vi "APX TMP control.vi"() -> ()   [LabVIEW 2015]
uses:
  <vilib>/Instr/_visa.llb/VISA Configure Serial Port (Instr).vi
  <userlib>/caLab/Private/Get_PV-1D.vi
  <userlib>/caLab/Private/Put_DBL-1D_PV-1D.vi
panel:
  out "Status":bool
  in  "stop":bool
  in  "APX:BPTurebo_ENB":bool
  in  "APX:GASTurbo_ENB":bool
  in  "APX:HPCTurbo_ENB":bool
  in  "APX:PREPTurbo_ENB":bool
  in  "APX:HEMTurbo_ENB":bool
  in  "APX:L2Turbo_ENB":bool
  in  "APX:AP2Turbo_ENB":bool
  in  "APX:AP1Turbo_ENB":bool
  out "APX:BPTurboS":dbl
  out "APX:BPTrubo_STOP":bool
  out "APX:BPTurbo_START":bool
  out "APX:BPTurboPort":refnum<visa-resource-name>="COM4"
  out "APX:BPTurboF":dbl caption="F_20/Hz"
  out "APX:BPTurboP":dbl caption="P_20/W"
  out "APX:BPTurboS:STR":string
  out "APX:GASTurboS":dbl
  out "APX:GASTurbo_STOP":bool
  out "APX:GASTurbo_START":bool
  out "APX:GASTurboPort":refnum<visa-resource-name>="COM4"
  out "APX:GASTurboF":dbl caption="F_20/Hz"
  out "APX:GASTurboP":dbl caption="P_20/W"
  out "APX:GASTurboS:STR":string
  out "APX:HPCTurboS":dbl
  out "APX:HPCTrubo_STOP":bool
  out "APX:HPCTurbo_START":bool
  out "APX:HPCTurboPort":refnum<visa-resource-name>="COM4"
  out "APX:HPCTurboF":dbl caption="F_20/Hz"
  out "APX:HPCTurboP":dbl caption="P_20/W"
  out "APX:HPCTurboS:STR":string
  out "APX:PREPTurboS":dbl
  out "APX:PREPTrubo_STOP":bool
  out "APX:PREPTurbo_START":bool
  out "APX:PREPTurboPort":refnum<visa-resource-name>="COM4"
  out "APX:PREPTurboF":dbl caption="F_20/Hz"
  out "APX:PREPTurboP":dbl caption="P_20/W"
  out "APX:PREPTurboS:STR":string
  out "APX:HEMTurboS":dbl
  out "APX:HEMTrubo_STOP":bool
  out "APX:HEMTurbo_START":bool
  out "APX:HEMTurboPort":refnum<visa-resource-name>="COM4"
  out "APX:HEMTurboF":dbl caption="F_20/Hz"
  out "APX:HEMTurboP":dbl caption="P_20/W"
  out "APX:HEMTurboS:STR":string
  out "APX:L2TurboS":dbl
  out "APX:L2Trubo_STOP":bool
  out "APX:L2Turbo_START":bool
  out "APX:L2TuroboPort":refnum<visa-resource-name>="COM4"
  out "APX:L2TurboF":dbl caption="F_20/Hz"
  out "APX:L2TurboP":dbl caption="P_20/W"
  out "APX:L2STurboS:STR":string
  out "APX:AP2TurboS":dbl
  out "APX:AP2Trubo_STOP":bool
  out "APX:AP2Turbo_START":bool
  out "APX:AP2TruboPort":refnum<visa-resource-name>="COM4"
  out "APX:AP2TurboF":dbl caption="F_20/Hz"
  out "APX:AP2TurboP":dbl caption="P_20/W"
  out "APX:AP2TurboS:STR":string
  out "APX:AP1STurboS":dbl
  out "APX:AP1Trubo_STOP":bool
  out "APX:APITurbo_START":bool
  out "APX:AP1TurboPort":refnum<visa-resource-name>="COM4"
  out "APX:AP1TurboF":dbl caption="F_20/Hz"
  out "APX:AP1TurboP":dbl caption="P_20/W"
  out "APX:AP1TurboS:STR":string
  # "APX Turbo"
  # "COM6"
  # "COM4"
  # "COM5"
  # "COM25"
  # "COM26"
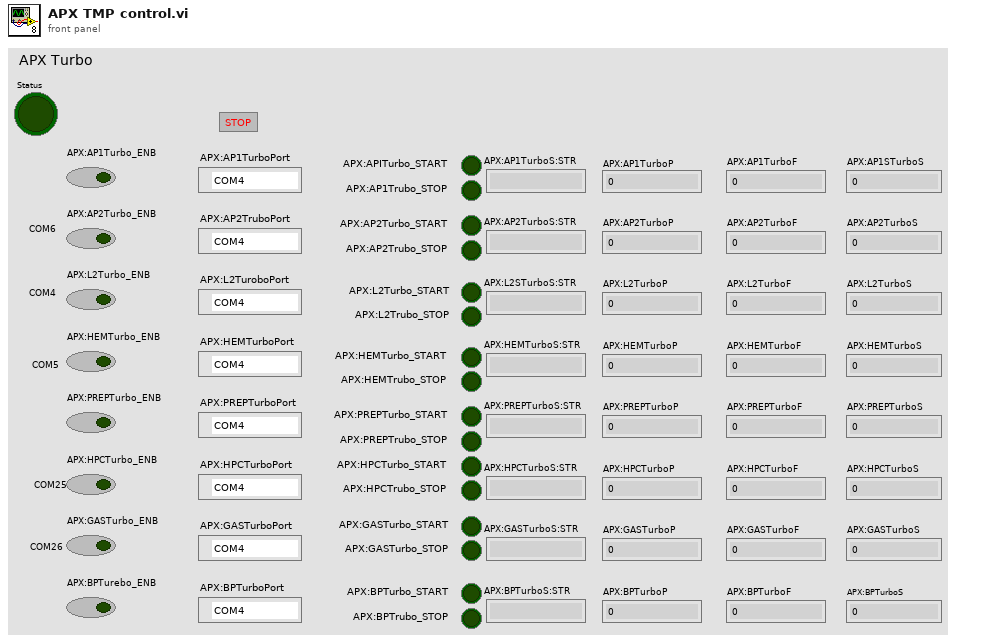
[diagram p1: front panel]
types:
  T1 = enum16{"START", "STOP", "REMOTE/SERIAL", "REMOTE", "SERIAL", "START/STOP", "PUMP STATUS", "Driving Frequency", "PUMP POWER", "PRESSURE"}
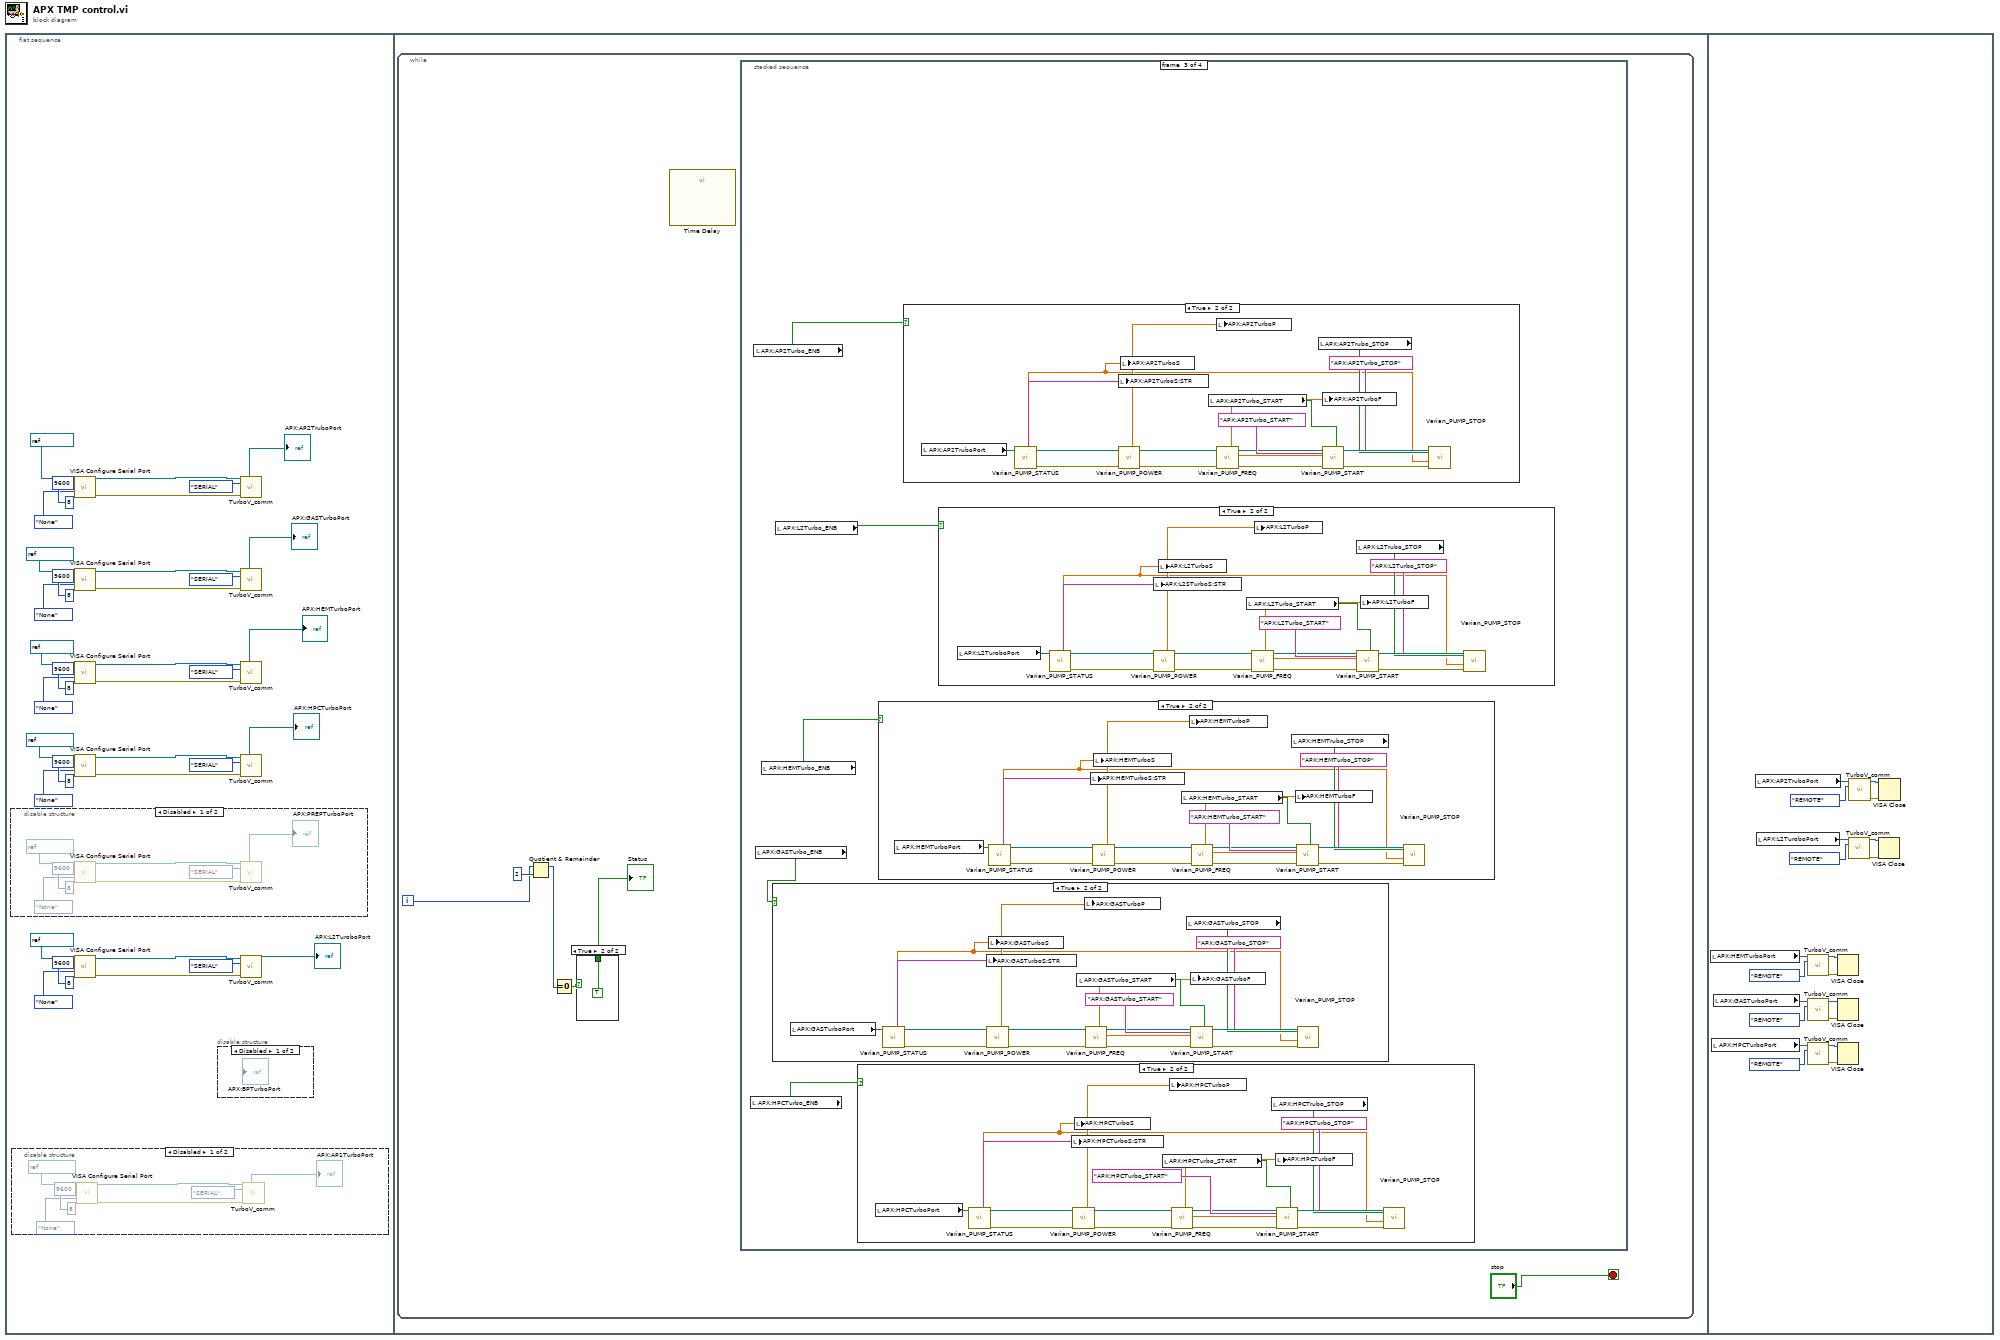
[diagram p0: block diagram]
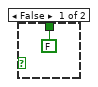
[diagram p5: hidden frame]
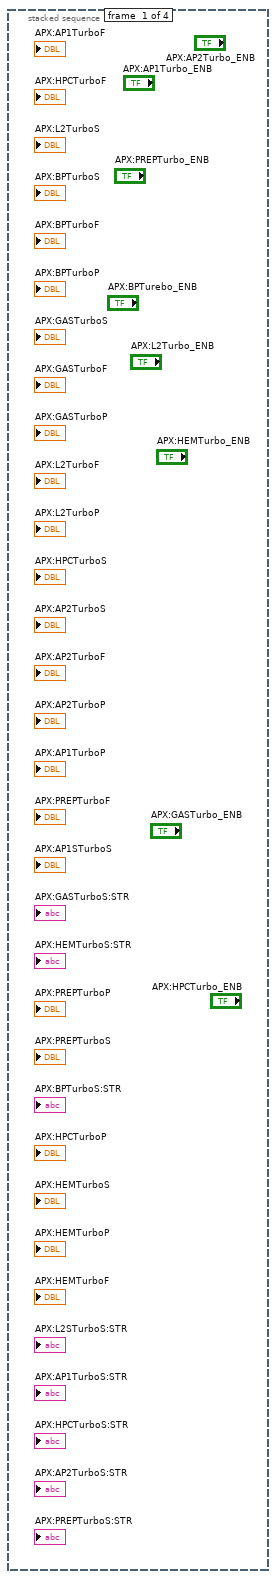
[diagram p6: hidden frame]
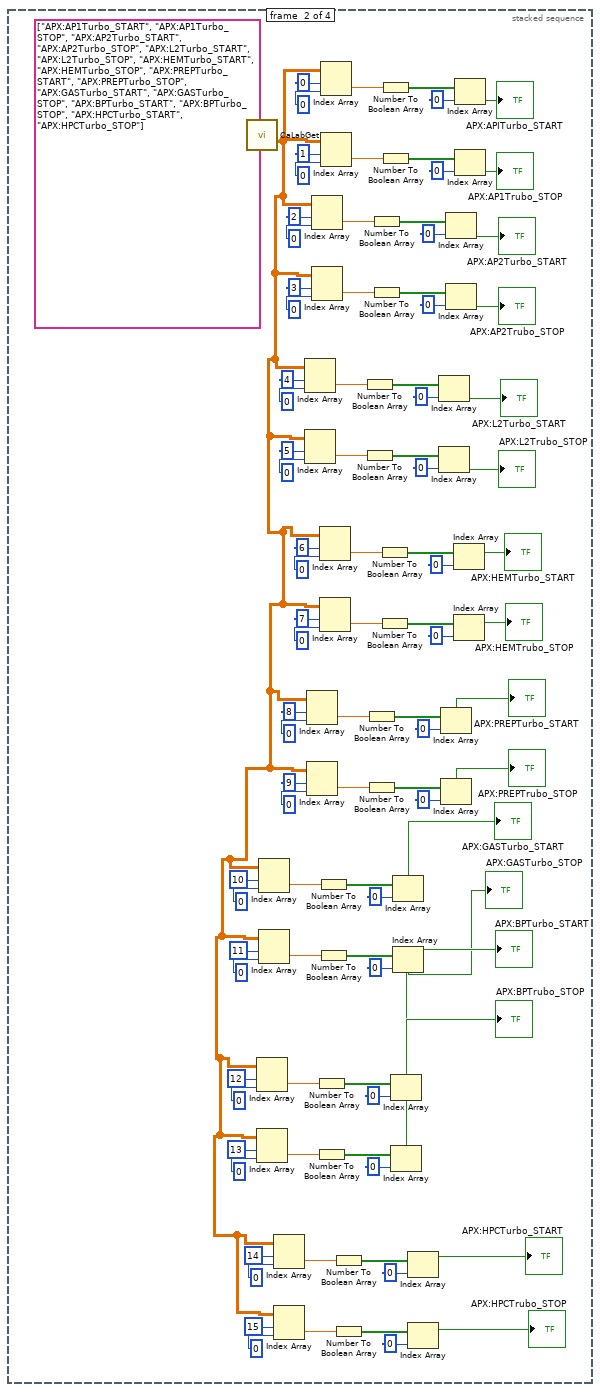
[diagram p7: hidden frame]
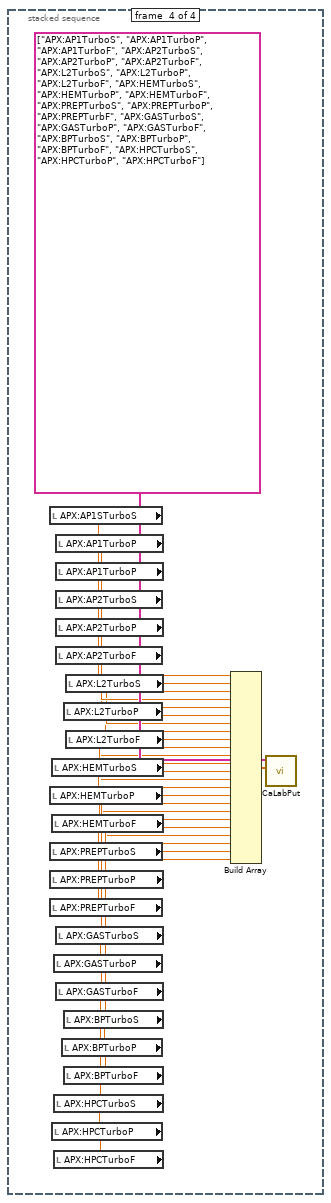
[diagram p13: hidden frame]
diagram:
  n1 = flat-sequence {
    frame #0 {
      n2 = disable-structure shown="Disabled" {
        frame Disabled {
          n3 = call-poly "VISA Configure Serial Port"("VISA resource name"=refnum<visa-resource-name> "COM26", "baud rate (9600)"=u32 9600, "data bits (8)"=u16 8, "parity (0:none)"=enum16{"None", "Odd", "Even", "Mark", "Space"}."None") -> ("VISA resource name out"=w53:refnum<visa-resource-name>, "error out"=w52:errorcluster)  [unwired: 10 in]
          n4 = call "TurboV_comm.vi"("VISA resource name"=w53, "Command"=T1."SERIAL", "error in (no error)"=w52) -> ("VISA resource name out"=→"APX:PREPTurboPort":refnum<visa-resource-name>)  [unwired: 10 in, 2 out]
        }
        frame Enabled {
        }
      }
      n5 = disable-structure shown="Disabled" {
        frame Disabled {
          n6 = call-poly "VISA Configure Serial Port"("VISA resource name"=refnum<visa-resource-name> "COM26", "baud rate (9600)"=u32 9600, "data bits (8)"=u16 8, "parity (0:none)"=enum16{"None", "Odd", "Even", "Mark", "Space"}."None") -> ("VISA resource name out"=w44:refnum<visa-resource-name>, "error out"=w43:errorcluster)  [unwired: 10 in]
          n7 = call "TurboV_comm.vi"("VISA resource name"=w44, "Command"=T1."SERIAL", "error in (no error)"=w43) -> ("VISA resource name out"=→"APX:AP1TurboPort":refnum<visa-resource-name>)  [unwired: 10 in, 2 out]
        }
        frame Enabled {
        }
      }
      n8 = call-poly "VISA Configure Serial Port"("VISA resource name"=refnum<visa-resource-name> "COM6", "baud rate (9600)"=u32 9600, "data bits (8)"=u16 8, "parity (0:none)"=enum16{"None", "Odd", "Even", "Mark", "Space"}."None") -> ("VISA resource name out"=w9:refnum<visa-resource-name>, "error out"=w8:errorcluster)  [unwired: 10 in]
      n9 = call-poly "VISA Configure Serial Port"("VISA resource name"=refnum<visa-resource-name> "COM26", "baud rate (9600)"=u32 9600, "data bits (8)"=u16 8, "parity (0:none)"=enum16{"None", "Odd", "Even", "Mark", "Space"}."None") -> ("VISA resource name out"=w16:refnum<visa-resource-name>, "error out"=w15:errorcluster)  [unwired: 10 in]
      n10 = call-poly "VISA Configure Serial Port"("VISA resource name"=refnum<visa-resource-name> "COM5", "baud rate (9600)"=u32 9600, "data bits (8)"=u16 8, "parity (0:none)"=enum16{"None", "Odd", "Even", "Mark", "Space"}."None") -> ("VISA resource name out"=w23:refnum<visa-resource-name>, "error out"=w22:errorcluster)  [unwired: 10 in]
      n11 = call-poly "VISA Configure Serial Port"("VISA resource name"=refnum<visa-resource-name> "COM25", "baud rate (9600)"=u32 9600, "data bits (8)"=u16 8, "parity (0:none)"=enum16{"None", "Odd", "Even", "Mark", "Space"}."None") -> ("VISA resource name out"=w30:refnum<visa-resource-name>, "error out"=w29:errorcluster)  [unwired: 10 in]
      n12 = call-poly "VISA Configure Serial Port"("VISA resource name"=refnum<visa-resource-name> "COM4", "baud rate (9600)"=u32 9600, "data bits (8)"=u16 8, "parity (0:none)"=enum16{"None", "Odd", "Even", "Mark", "Space"}."None") -> ("VISA resource name out"=w37:refnum<visa-resource-name>, "error out"=w36:errorcluster)  [unwired: 10 in]
      n13 = disable-structure shown="Disabled" {
        frame Disabled {
        }
        frame Enabled {
        }
      }
      n14 = call "TurboV_comm.vi"("VISA resource name"=w9, "Command"=T1."SERIAL", "error in (no error)"=w8) -> ("VISA resource name out"=→"APX:AP2TruboPort":refnum<visa-resource-name>)  [unwired: 10 in, 2 out]
      n15 = call "TurboV_comm.vi"("VISA resource name"=w16, "Command"=T1."SERIAL", "error in (no error)"=w15) -> ("VISA resource name out"=→"APX:GASTurboPort":refnum<visa-resource-name>)  [unwired: 10 in, 2 out]
      n16 = call "TurboV_comm.vi"("VISA resource name"=w23, "Command"=T1."SERIAL", "error in (no error)"=w22) -> ("VISA resource name out"=→"APX:HEMTurboPort":refnum<visa-resource-name>)  [unwired: 10 in, 2 out]
      n17 = call "TurboV_comm.vi"("VISA resource name"=w30, "Command"=T1."SERIAL", "error in (no error)"=w29) -> ("VISA resource name out"=→"APX:HPCTurboPort":refnum<visa-resource-name>)  [unwired: 10 in, 2 out]
      n18 = call "TurboV_comm.vi"("VISA resource name"=w37, "Command"=T1."SERIAL", "error in (no error)"=w36) -> ("VISA resource name out"=→"APX:L2TuroboPort":refnum<visa-resource-name>)  [unwired: 10 in, 2 out]
    }
    frame #1 {
      n19 = while {
        i -> [w58]
        stop <- "stop" stop-if-true
        n20 = Quotient & Remainder(x=w58, y=2) -> (x-y*floor(x/y)=w60:i32)  [unwired: 1 out]
        n21 = Equal To 0?(x=w60) -> (x = 0?=w61:bool)
        n22 = case shown="True" w61 {
          tunnel: [FALSE ("Status") TRUE ("Status")] -> w57
          frame False {
          }
          frame True {
          }
        }
        "Status" <- w57
        n23 = call "Time Delay"() -> ()  [unwired: 11 in, 1 out]
        n24 = stacked-sequence {
          frame #0 {
          }
          frame #1 {
            n25 = call-poly "CaLabGet.vi"("PV Names"=string[] ["APX:AP1Turbo_START", "APX:AP1Turbo_STOP", "APX:AP2Turbo_START", "APX:AP2Turbo_STOP", "APX:L2Turbo_START", "APX:L2Turbo_STOP", "APX:HEMTurbo_START", "APX:HEMTurbo_STOP", "APX:PREPTurbo_START", "APX:PREPTurbo_STOP", "APX:GASTurbo_START", "APX:GASTurbo_STOP", "APX:BPTurbo_START", "APX:BPTurbo_STOP", "APX:HPCTurbo_START", "APX:HPCTurbo_STOP"]) -> ("Value Array (number)"=w160:dbl[][])  [unwired: 8 in, 6 out]
            n26 = Index Array(array=w160, index (row)=12 ("disabled index (row)"), index (col)=0 ("index (row)")) -> (element=w142:dbl)
            n27 = Index Array(array=w160, index (row)=13 ("disabled index (row)"), index (col)=0 ("index (row)")) -> (element=w147:dbl)
            n28 = Index Array(array=w160, index (row)=10 ("disabled index (row)"), index (col)=0 ("index (row)")) -> (element=w130:dbl)
            n29 = Index Array(array=w160, index (row)=11 ("disabled index (row)"), index (col)=0 ("index (row)")) -> (element=w135:dbl)
            n30 = Index Array(array=w160, index (row)=14 ("disabled index (row)"), index (col)=0 ("index (row)")) -> (element=w154:dbl)
            n31 = Index Array(array=w160, index (row)=15 ("disabled index (row)"), index (col)=0 ("index (row)")) -> (element=w159:dbl)
            n32 = Index Array(array=w160, index (row)=4 ("disabled index (row)"), index (col)=0 ("index (row)")) -> (element=w94:dbl)
            n33 = Index Array(array=w160, index (row)=5 ("disabled index (row)"), index (col)=0 ("index (row)")) -> (element=w99:dbl)
            n34 = Index Array(array=w160, index (row)=8 ("disabled index (row)"), index (col)=0 ("index (row)")) -> (element=w118:dbl)
            n35 = Index Array(array=w160, index (row)=9 ("disabled index (row)"), index (col)=0 ("index (row)")) -> (element=w123:dbl)
            n36 = Index Array(array=w160, index (row)=2 ("disabled index (row)"), index (col)=0 ("index (row)")) -> (element=w82:dbl)
            n37 = Index Array(array=w160, index (row)=3 ("disabled index (row)"), index (col)=0 ("index (row)")) -> (element=w87:dbl)
            n38 = Number To Boolean Array(number=w142) -> (Boolean array=w140:bool[])
            n39 = Number To Boolean Array(number=w147) -> (Boolean array=w145:bool[])
            n40 = Number To Boolean Array(number=w130) -> (Boolean array=w128:bool[])
            n41 = Number To Boolean Array(number=w135) -> (Boolean array=w133:bool[])
            n42 = Index Array(array=w160, index (row)=6 ("disabled index (row)"), index (col)=0 ("index (row)")) -> (element=w106:dbl)
            n43 = Index Array(array=w160, index (row)=7 ("disabled index (row)"), index (col)=0 ("index (row)")) -> (element=w111:dbl)
            n44 = Index Array(array=w160, index (row)=0 ("disabled index (row)"), index (col)=0 ("index (row)")) -> (element=w70:dbl)
            n45 = Index Array(array=w160, index (row)=1 ("disabled index (row)"), index (col)=0 ("index (row)")) -> (element=w75:dbl)
            n46 = Number To Boolean Array(number=w154) -> (Boolean array=w152:bool[])
            n47 = Number To Boolean Array(number=w159) -> (Boolean array=w157:bool[])
            n48 = Number To Boolean Array(number=w94) -> (Boolean array=w92:bool[])
            n49 = Number To Boolean Array(number=w99) -> (Boolean array=w97:bool[])
            n50 = Number To Boolean Array(number=w118) -> (Boolean array=w116:bool[])
            n51 = Number To Boolean Array(number=w123) -> (Boolean array=w121:bool[])
            n52 = Number To Boolean Array(number=w82) -> (Boolean array=w80:bool[])
            n53 = Number To Boolean Array(number=w87) -> (Boolean array=w85:bool[])
            n54 = Number To Boolean Array(number=w106) -> (Boolean array=w104:bool[])
            n55 = Number To Boolean Array(number=w111) -> (Boolean array=w109:bool[])
            n56 = Number To Boolean Array(number=w70) -> (Boolean array=w68:bool[])
            n57 = Number To Boolean Array(number=w75) -> (Boolean array=w73:bool[])
            n58 = Index Array(array=w140, index=0) -> (element=→"APX:BPTurbo_START":bool)
            n59 = Index Array(array=w145, index=0) -> (element=→"APX:BPTrubo_STOP":bool)
            n60 = Index Array(array=w128, index=0) -> (element=→"APX:GASTurbo_START":bool)
            n61 = Index Array(array=w133, index=0) -> (element=→"APX:GASTurbo_STOP":bool)
            n62 = Index Array(array=w152, index=0) -> (element=→"APX:HPCTurbo_START":bool)
            n63 = Index Array(array=w157, index=0) -> (element=→"APX:HPCTrubo_STOP":bool)
            n64 = Index Array(array=w92, index=0) -> (element=→"APX:L2Turbo_START":bool)
            n65 = Index Array(array=w97, index=0) -> (element=→"APX:L2Trubo_STOP":bool)
            n66 = Index Array(array=w116, index=0) -> (element=→"APX:PREPTurbo_START":bool)
            n67 = Index Array(array=w121, index=0) -> (element=→"APX:PREPTrubo_STOP":bool)
            n68 = Index Array(array=w80, index=0) -> (element=→"APX:AP2Turbo_START":bool)
            n69 = Index Array(array=w85, index=0) -> (element=→"APX:AP2Trubo_STOP":bool)
            n70 = Index Array(array=w104, index=0) -> (element=→"APX:HEMTurbo_START":bool)
            n71 = Index Array(array=w109, index=0) -> (element=→"APX:HEMTrubo_STOP":bool)
            n72 = Index Array(array=w68, index=0) -> (element=→"APX:APITurbo_START":bool)
            n73 = Index Array(array=w73, index=0) -> (element=→"APX:AP1Trubo_STOP":bool)
          }
          frame #2 {
            n74 = local read "APX:HPCTurbo_ENB"() -> (w163:bool)
            n75 = local read "APX:AP2Turbo_ENB"() -> (w167:bool)
            n76 = local read "APX:GASTurbo_ENB"() -> (w164:bool)
            n77 = local read "APX:HEMTurbo_ENB"() -> (w165:bool)
            n78 = case shown="True" w164 {
              frame False {
              }
              frame True {
                n79 = local read "APX:GASTurboPort"() -> (w195:refnum<visa-resource-name>)
                n80 = call "Varian_PUMP_STATUS.vi"("VISA Refnum in"=w195) -> ("error out"=w196:errorcluster, "String"=w201:string, "Numeric"=w185:dbl, "VISA Refnum out"=w200:refnum<visa-resource-name>)  [unwired: 7 in]
                n81 = local write "APX:GASTurboS:STR"(w201) -> ()
                n82 = call "Varian_PUMP_POWER.vi"("error in (no error)"=w196, "VISA Refnum in"=w200) -> ("error out"=w197:errorcluster, "Numeric"=w199:dbl, "VISA Refnum out"=w198:refnum<visa-resource-name>)  [unwired: 7 in]
                n83 = local write "APX:GASTurboS"(w185) -> ()
                n84 = local read "APX:GASTurbo_START"() -> (w193:bool)
                n85 = local write "APX:GASTurboP"(w199) -> ()
                n86 = call "Varian_PUMP_FREQ.vi"("error in (no error)"=w197, "VISA Refnum in"=w198) -> ("error out"=w189:errorcluster, "Numeric"=w190:dbl, "VISA Refnum out"=w191:refnum<visa-resource-name>)  [unwired: 7 in]
                n87 = local read "APX:GASTurbo_STOP"() -> (w188:bool)
                n88 = local write "APX:GASTurboF"(w190) -> ()
                n89 = call "Varian_PUMP_START.vi"("APX:APITurbo_START"=w193, "PV Name"="APX:GASTurbo_START", "error in"=w189, "APX:AP1TurboF"=w190, "VISA Refnum in"=w191) -> ("error out"=w186:errorcluster, "VISA Refnum out"=w194:refnum<visa-resource-name>)  [unwired: 5 in]
                n90 = call "Varian_PUMP_STOP.vi"("APX:AP1Trubo_STOP"=w188, "PV Name"="APX:GASTurbo_STOP", "error in (no error)"=w186, "APX:AP1STurboS"=w185, "VISA Refnum in"=w194) -> ()  [unwired: 5 in, 2 out]
              }
            }
            n91 = local read "APX:L2Turbo_ENB"() -> (w166:bool)
            n92 = case shown="True" w163 {
              frame False {
              }
              frame True {
                n93 = local read "APX:HPCTurboPort"() -> (w178:refnum<visa-resource-name>)
                n94 = call "Varian_PUMP_STATUS.vi"("VISA Refnum in"=w178) -> ("error out"=w179:errorcluster, "String"=w184:string, "Numeric"=w168:dbl, "VISA Refnum out"=w183:refnum<visa-resource-name>)  [unwired: 7 in]
                n95 = local write "APX:HPCTurboS:STR"(w184) -> ()
                n96 = call "Varian_PUMP_POWER.vi"("error in (no error)"=w179, "VISA Refnum in"=w183) -> ("error out"=w180:errorcluster, "Numeric"=w182:dbl, "VISA Refnum out"=w181:refnum<visa-resource-name>)  [unwired: 7 in]
                n97 = local write "APX:HPCTurboS"(w168) -> ()
                n98 = local read "APX:HPCTurbo_START"() -> (w176:bool)
                n99 = local write "APX:HPCTurboP"(w182) -> ()
                n100 = call "Varian_PUMP_FREQ.vi"("error in (no error)"=w180, "VISA Refnum in"=w181) -> ("error out"=w172:errorcluster, "Numeric"=w173:dbl, "VISA Refnum out"=w174:refnum<visa-resource-name>)  [unwired: 7 in]
                n101 = local read "APX:HPCTrubo_STOP"() -> (w171:bool)
                n102 = local write "APX:HPCTurboF"(w173) -> ()
                n103 = call "Varian_PUMP_START.vi"("APX:APITurbo_START"=w176, "PV Name"="APX:HPCTurbo_START", "error in"=w172, "APX:AP1TurboF"=w173, "VISA Refnum in"=w174) -> ("error out"=w169:errorcluster, "VISA Refnum out"=w177:refnum<visa-resource-name>)  [unwired: 5 in]
                n104 = call "Varian_PUMP_STOP.vi"("APX:AP1Trubo_STOP"=w171, "PV Name"="APX:HPCTurbo_STOP", "error in (no error)"=w169, "APX:AP1STurboS"=w168, "VISA Refnum in"=w177) -> ()  [unwired: 5 in, 2 out]
              }
            }
            n105 = case shown="True" w165 {
              frame False {
              }
              frame True {
                n106 = local read "APX:HEMTurboPort"() -> (w212:refnum<visa-resource-name>)
                n107 = call "Varian_PUMP_STATUS.vi"("VISA Refnum in"=w212) -> ("error out"=w213:errorcluster, "String"=w218:string, "Numeric"=w202:dbl, "VISA Refnum out"=w217:refnum<visa-resource-name>)  [unwired: 7 in]
                n108 = local write "APX:HEMTurboS:STR"(w218) -> ()
                n109 = call "Varian_PUMP_POWER.vi"("error in (no error)"=w213, "VISA Refnum in"=w217) -> ("error out"=w214:errorcluster, "Numeric"=w216:dbl, "VISA Refnum out"=w215:refnum<visa-resource-name>)  [unwired: 7 in]
                n110 = local write "APX:HEMTurboS"(w202) -> ()
                n111 = local read "APX:HEMTurbo_START"() -> (w210:bool)
                n112 = local write "APX:HEMTurboP"(w216) -> ()
                n113 = call "Varian_PUMP_FREQ.vi"("error in (no error)"=w214, "VISA Refnum in"=w215) -> ("error out"=w206:errorcluster, "Numeric"=w207:dbl, "VISA Refnum out"=w208:refnum<visa-resource-name>)  [unwired: 7 in]
                n114 = local read "APX:HEMTrubo_STOP"() -> (w205:bool)
                n115 = local write "APX:HEMTurboF"(w207) -> ()
                n116 = call "Varian_PUMP_START.vi"("APX:APITurbo_START"=w210, "PV Name"="APX:HEMTurbo_START", "error in"=w206, "APX:AP1TurboF"=w207, "VISA Refnum in"=w208) -> ("error out"=w203:errorcluster, "VISA Refnum out"=w211:refnum<visa-resource-name>)  [unwired: 5 in]
                n117 = call "Varian_PUMP_STOP.vi"("APX:AP1Trubo_STOP"=w205, "PV Name"="APX:HEMTurbo_STOP", "error in (no error)"=w203, "APX:AP1STurboS"=w202, "VISA Refnum in"=w211) -> ()  [unwired: 5 in, 2 out]
              }
            }
            n118 = case shown="True" w167 {
              frame False {
              }
              frame True {
                n119 = local read "APX:AP2TruboPort"() -> (w246:refnum<visa-resource-name>)
                n120 = call "Varian_PUMP_STATUS.vi"("VISA Refnum in"=w246) -> ("error out"=w247:errorcluster, "String"=w252:string, "Numeric"=w236:dbl, "VISA Refnum out"=w251:refnum<visa-resource-name>)  [unwired: 7 in]
                n121 = local write "APX:AP2TurboS:STR"(w252) -> ()
                n122 = call "Varian_PUMP_POWER.vi"("error in (no error)"=w247, "VISA Refnum in"=w251) -> ("error out"=w248:errorcluster, "Numeric"=w250:dbl, "VISA Refnum out"=w249:refnum<visa-resource-name>)  [unwired: 7 in]
                n123 = local write "APX:AP2TurboS"(w236) -> ()
                n124 = local read "APX:AP2Turbo_START"() -> (w244:bool)
                n125 = local write "APX:AP2TurboP"(w250) -> ()
                n126 = call "Varian_PUMP_FREQ.vi"("error in (no error)"=w248, "VISA Refnum in"=w249) -> ("error out"=w240:errorcluster, "Numeric"=w241:dbl, "VISA Refnum out"=w242:refnum<visa-resource-name>)  [unwired: 7 in]
                n127 = local read "APX:AP2Trubo_STOP"() -> (w239:bool)
                n128 = local write "APX:AP2TurboF"(w241) -> ()
                n129 = call "Varian_PUMP_START.vi"("APX:APITurbo_START"=w244, "PV Name"="APX:AP2Turbo_START", "error in"=w240, "APX:AP1TurboF"=w241, "VISA Refnum in"=w242) -> ("error out"=w237:errorcluster, "VISA Refnum out"=w245:refnum<visa-resource-name>)  [unwired: 5 in]
                n130 = call "Varian_PUMP_STOP.vi"("APX:AP1Trubo_STOP"=w239, "PV Name"="APX:AP2Turbo_STOP", "error in (no error)"=w237, "APX:AP1STurboS"=w236, "VISA Refnum in"=w245) -> ()  [unwired: 5 in, 2 out]
              }
            }
            n131 = case shown="True" w166 {
              frame False {
              }
              frame True {
                n132 = local read "APX:L2TuroboPort"() -> (w229:refnum<visa-resource-name>)
                n133 = call "Varian_PUMP_STATUS.vi"("VISA Refnum in"=w229) -> ("error out"=w230:errorcluster, "String"=w235:string, "Numeric"=w219:dbl, "VISA Refnum out"=w234:refnum<visa-resource-name>)  [unwired: 7 in]
                n134 = call "Varian_PUMP_POWER.vi"("error in (no error)"=w230, "VISA Refnum in"=w234) -> ("error out"=w231:errorcluster, "Numeric"=w233:dbl, "VISA Refnum out"=w232:refnum<visa-resource-name>)  [unwired: 7 in]
                n135 = local write "APX:L2STurboS:STR"(w235) -> ()
                n136 = local write "APX:L2TurboS"(w219) -> ()
                n137 = local read "APX:L2Turbo_START"() -> (w227:bool)
                n138 = call "Varian_PUMP_FREQ.vi"("error in (no error)"=w231, "VISA Refnum in"=w232) -> ("error out"=w223:errorcluster, "Numeric"=w224:dbl, "VISA Refnum out"=w225:refnum<visa-resource-name>)  [unwired: 7 in]
                n139 = local write "APX:L2TurboP"(w233) -> ()
                n140 = local read "APX:L2Trubo_STOP"() -> (w222:bool)
                n141 = call "Varian_PUMP_START.vi"("APX:APITurbo_START"=w227, "PV Name"="APX:L2Turbo_START", "error in"=w223, "APX:AP1TurboF"=w224, "VISA Refnum in"=w225) -> ("error out"=w220:errorcluster, "VISA Refnum out"=w228:refnum<visa-resource-name>)  [unwired: 5 in]
                n142 = local write "APX:L2TurboF"(w224) -> ()
                n143 = call "Varian_PUMP_STOP.vi"("APX:AP1Trubo_STOP"=w222, "PV Name"="APX:L2Turbo_STOP", "error in (no error)"=w220, "APX:AP1STurboS"=w219, "VISA Refnum in"=w228) -> ()  [unwired: 5 in, 2 out]
              }
            }
          }
          frame #3 {
            n144 = local read "APX:AP1STurboS"() -> (w275:dbl)
            n145 = local read "APX:HEMTurboP"() -> (w266:dbl)
            n146 = local read "APX:PREPTurboS"() -> (w264:dbl)
            n147 = local read "APX:PREPTurboP"() -> (w263:dbl)
            n148 = local read "APX:PREPTurboF"() -> (w262:dbl)
            n149 = local read "APX:HEMTurboS"() -> (w267:dbl)
            n150 = local read "APX:HEMTurboF"() -> (w265:dbl)
            n151 = local read "APX:HPCTurboP"() -> (w254:dbl)
            n152 = local read "APX:GASTurboP"() -> (w260:dbl)
            n153 = local read "APX:HPCTurboS"() -> (w255:dbl)
            n154 = local read "APX:HPCTurboF"() -> (w253:dbl)
            n155 = local read "APX:AP1TurboP"() -> (w276:dbl)
            n156 = local read "APX:AP1TurboP"() -> (w274:dbl)
            n157 = local read "APX:AP2TurboS"() -> (w273:dbl)
            n158 = local read "APX:AP2TurboP"() -> (w272:dbl)
            n159 = local read "APX:AP2TurboF"() -> (w271:dbl)
            n160 = local read "APX:GASTurboS"() -> (w261:dbl)
            n161 = local read "APX:GASTurboF"() -> (w259:dbl)
            n162 = local read "APX:BPTurboP"() -> (w257:dbl)
            n163 = local read "APX:L2TurboP"() -> (w269:dbl)
            n164 = local read "APX:BPTurboS"() -> (w258:dbl)
            n165 = local read "APX:BPTurboF"() -> (w256:dbl)
            n166 = local read "APX:L2TurboS"() -> (w270:dbl)
            n167 = local read "APX:L2TurboF"() -> (w268:dbl)
            n168 = Build Array(w275, w276, w274, w273, w272, w271, w270, w269, w268, w267, w266, w265, w264, w263, w262, w261, w260, w259, w258, w257, w256, w255, w254, w253) -> (w277:dbl[])
            n169 = call-poly <userlib>:"CaLabPut.vi"("Values"=w277, "PV Names"=string[] ["APX:AP1TurboS", "APX:AP1TurboP", "APX:AP1TurboF", "APX:AP2TurboS", "APX:AP2TurboP", "APX:AP2TurboF", "APX:L2TurboS", "APX:L2TurboP", "APX:L2TurboF", "APX:HEMTurboS", "APX:HEMTurboP", "APX:HEMTurboF", "APX:PREPTurboS", "APX:PREPTurboP", "APX:PREPTurbF", "APX:GASTurboS", "APX:GASTurboP", "APX:GASTurboF", "APX:BPTurboS", "APX:BPTurboP", "APX:BPTurboF", "APX:HPCTurboS", "APX:HPCTurboP", "APX:HPCTurboF"]) -> ()  [unwired: 6 in, 4 out]
          }
        }
      }
    }
    frame #2 {
      n170 = local read "APX:HEMTurboPort"() -> (w281:refnum<visa-resource-name>)
      n171 = local read "APX:HPCTurboPort"() -> (w279:refnum<visa-resource-name>)
      n172 = local read "APX:GASTurboPort"() -> (w280:refnum<visa-resource-name>)
      n173 = local read "APX:AP2TruboPort"() -> (w283:refnum<visa-resource-name>)
      n174 = local read "APX:L2TuroboPort"() -> (w282:refnum<visa-resource-name>)
      n175 = call "TurboV_comm.vi"("VISA resource name"=w281, "Command"=T1."REMOTE") -> ("VISA resource name out"=w291:refnum<visa-resource-name>, "error out"=w290:errorcluster)  [unwired: 11 in, 1 out]
      n176 = call "TurboV_comm.vi"("VISA resource name"=w280, "Command"=T1."REMOTE") -> ("VISA resource name out"=w288:refnum<visa-resource-name>, "error out"=w287:errorcluster)  [unwired: 11 in, 1 out]
      n177 = call "TurboV_comm.vi"("VISA resource name"=w279, "Command"=T1."REMOTE") -> ("VISA resource name out"=w285:refnum<visa-resource-name>, "error out"=w284:errorcluster)  [unwired: 11 in, 1 out]
      n178 = VISA Close(VISA resource name=w291, error in (no error)=w290) -> ()  [unwired: 1 out]
      n179 = VISA Close(VISA resource name=w288, error in (no error)=w287) -> ()  [unwired: 1 out]
      n180 = VISA Close(VISA resource name=w285, error in (no error)=w284) -> ()  [unwired: 1 out]
      n181 = call "TurboV_comm.vi"("VISA resource name"=w282, "Command"=T1."REMOTE") -> ("VISA resource name out"=w294:refnum<visa-resource-name>, "error out"=w293:errorcluster)  [unwired: 11 in, 1 out]
      n182 = call "TurboV_comm.vi"("VISA resource name"=w283, "Command"=T1."REMOTE") -> ("VISA resource name out"=w297:refnum<visa-resource-name>, "error out"=w296:errorcluster)  [unwired: 11 in, 1 out]
      n183 = VISA Close(VISA resource name=w294, error in (no error)=w293) -> ()  [unwired: 1 out]
      n184 = VISA Close(VISA resource name=w297, error in (no error)=w296) -> ()  [unwired: 1 out]
    }
  }
